vi "Write RS232Config.vi"(10 "RS232Config":T1={"VISA resource name"="", "Baud Rate"=9600, "Data Bits"=8, "Parity"=enum."None", "Stop Bits"=10, "Flow Control"=0, "Timeout (ms)"=10000} {"Stop Bits" items=["1.0"=10, "1.5"=15, "2.0"=20]; "Flow Control" items=["None", "XON/XOFF", "RTS/CTS", "XON/XOFF & RTS/CTS", "DTR/DSR", "XON/XOFF & DTR/DSR"]; "Data Bits" min=5 max=8 step=1}, 11 "RS232 in":refnum<class "RS232.lvclass">) -> (3 "RS232 out":refnum<class "RS232.lvclass">)   [LabVIEW 2012, in "RS232.lvclass"]
uses:
  RS232.lvclass
  Configuration/RS232Config.ctl
  RS232.lvclass/RS232.ctl
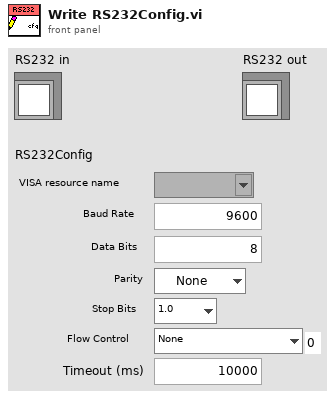
[diagram p1: front panel]
types:
  T1 = typedef "RS232Config.ctl" = cluster{"VISA resource name":refnum<visa-resource-name>, "Baud Rate":u32, "Data Bits":u16, "Parity":enum16{"None", "Odd", "Even", "Mark", "Space"}, "Stop Bits":u16, "Flow Control":u16, "Timeout (ms)":u32}
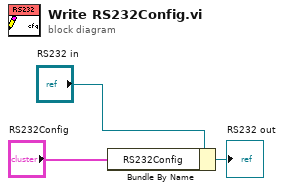
[diagram p0: block diagram]
diagram:
  n1 = Bundle By Name(cluster="RS232 in", "RS232Config"="RS232Config") -> (→"RS232 out":refnum<class "RS232.lvclass">)
